vi "Scroll_init.vi"(7 "Sum":u32, 8 "error in (no error)":errorcluster, 9 "Index":u32, 10 "Scroll":refnum<vi>, 11 "Scroller in":refnum<class "Scroller.lvclass">) -> (0 "error out":errorcluster, 3 "Scroller out":refnum<class "Scroller.lvclass">)   [LabVIEW 2015, in "ActorManagement.lvlib" / "Scroller.lvclass"]
uses:
  Scroller.lvclass
  Config/g_tabSetting.vi
  ActorManagement.lvlib
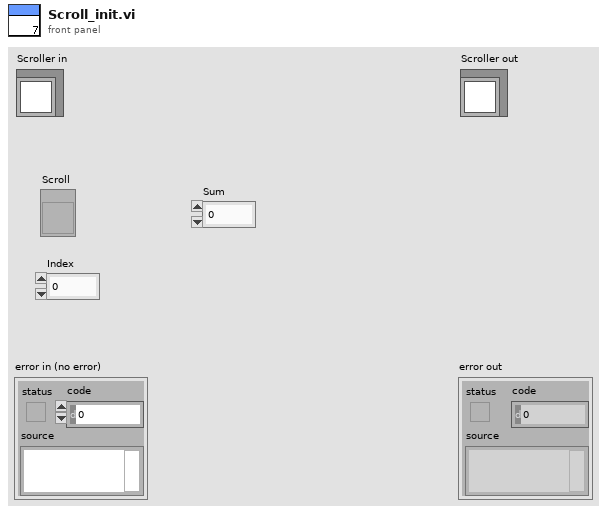
[diagram p1: front panel]
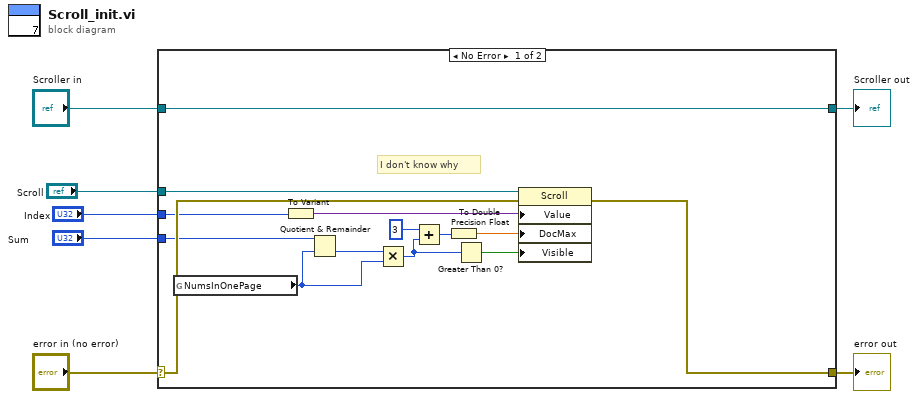
[diagram p0: block diagram]
diagram:
  n1 = case shown="No Error" "error in (no error)" {
    selector: "error in (no error)" -> [w19 w23]
    tunnel: [w15 w23] -> w6
    tunnel: [w21 w22] -> w4
    tunnel: "Scroller in" -> [w21 w22]
    tunnel: "Scroll" -> [w20 _]
    tunnel: "Index" -> [w18 _]
    tunnel: "Sum" -> [w14 _]
    frame No Error {
      # "I don't know why"
      n2 = global read "g_tabSetting.vi" "NumsInOnePage"() -> (w12:u32)
      n3 = To Variant(anything=w18) -> (Variant=w17:variant)
      n4 = Quotient & Remainder(x=w14, y=w12) -> (floor(x/y)=w13:u32)  [unwired: 1 out]
      n5 = Multiply(x=w13, y=w12) -> (x*y=w10:u32)
      n6 = Add(x=u32 3, y=w10) -> (x+y=w8:u32)
      n7 = To Double Precision Float(number=w8) -> (double precision float=w16:dbl)
      n8 = Greater Than 0?(x=w10) -> (x > 0?=w11:bool)
      n9 = property class="Scroll"(reference=w20, error in=w19, "Value"=w17, "DocMax"=w16, "Visible"=w11) -> (error out=w15:errorcluster)  [unwired: 1 out]
    }
    frame Error {
    }
  }
  "error out" <- w6
  "Scroller out" <- w4
